vi "final code.vi"() -> ()   [LabVIEW 2018]
uses:
  <vilib>/Analysis/Matrix/Datatypes/RealMatrix.ctl
  <vilib>/Analysis/Matrix/NI_Matrix.lvlib
panel:
  in  "Y":dbl(slide)=1.5703016241299301 scale=1.6..-1.6
  in  "X":dbl(slide)=-1.504382470119522 scale=-1.6..1.6
  out "3D Picture":refnum<vi>(3d-picture)
  in  "stop":bool
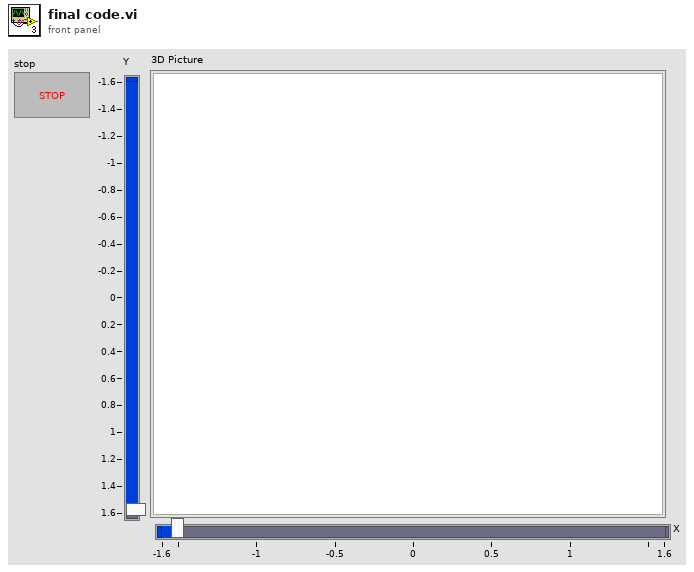
[diagram p1: front panel]
types:
  T1 = cluster{"Line width":sgl, "Line Color":u32, "Axes?":bool}
  T2 = typedef "NI_Matrix.lvlib/RealMatrix.ctl" = dbl[][]
  T3 = cluster{"Theta":dbl, "d":dbl, "a":dbl, "alpha (degrees)":dbl}[]
  T4 = cluster{"Theta":dbl, "d":dbl, "a":dbl, "alpha (degrees)":dbl}
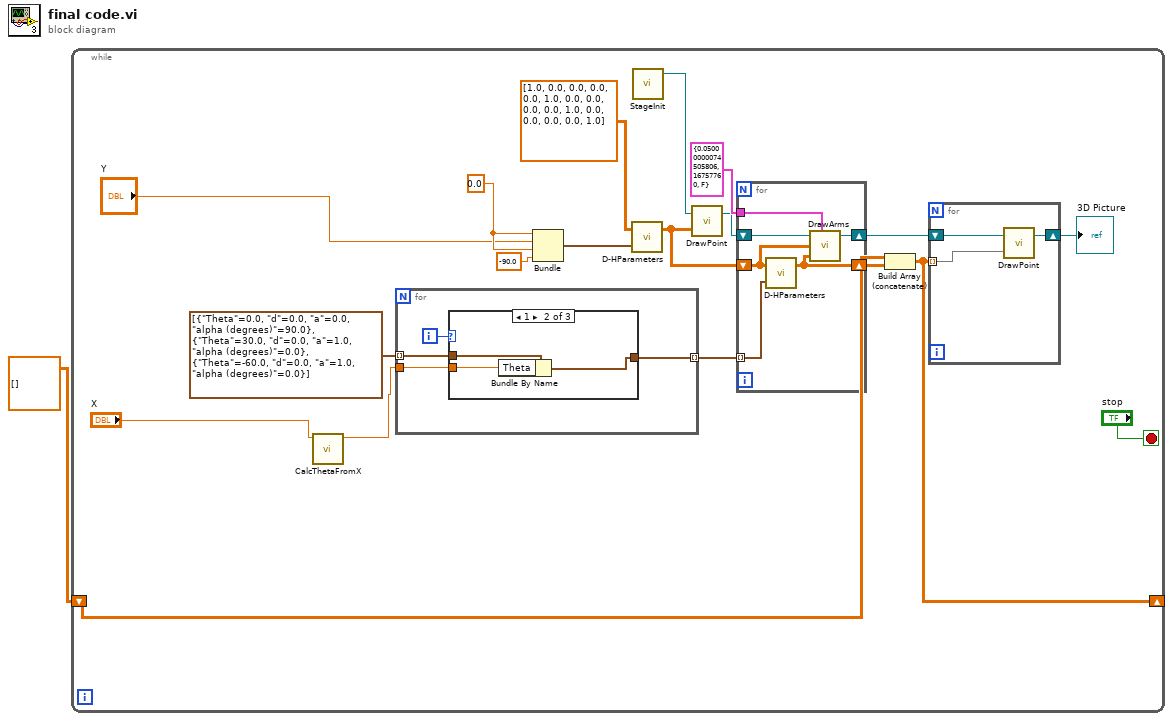
[diagram p0: block diagram]
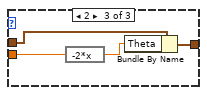
[diagram p3: hidden frame]
diagram:
  n1 = while {
    shift-right: [w19] -> _
    shift-left: dbl[][][] [] -> [w20]
    stop <- "stop" stop-if-true
    w5 = 0.0
    n2 = call "CalcThetaFromX.vi"("X"="X") -> ("Numeric"=w2:dbl)  [unwired: 10 in]
    n3 = for {
      tunnel: T3 [{"Theta"=0.0, "d"=0.0, "a"=0.0, "alpha (degrees)"=90.0}, {"Theta"=30.0, "d"=0.0, "a"=1.0, "alpha (degrees)"=0.0}, {"Theta"=-60.0, "d"=0.0, "a"=1.0, "alpha (degrees)"=0.0}] ("Joints") -> [w32] mode=indexing
      tunnel: [w31] -> w14 mode=indexing
      tunnel: w2 -> [w30]
      i -> [w33]
      n4 = case shown="1" w33 {
        tunnel: w32 -> [w34 w37 w41]
        tunnel: [w34 w36 w40] -> w31
        tunnel: w30 -> [_ w35 w39]
        frame 0, Default {
        }
        frame 1 {
          n5 = Bundle By Name(cluster=w37, "Theta"=w35) -> (w36:T4)
        }
        frame 2 {
          n6 = expression code="-2*x"(w39) -> (w38:dbl)
          n7 = Bundle By Name(cluster=w41, "Theta"=w38) -> (w40:T4)
        }
      }
    }
    n8 = Bundle(w5, "Y"="Y", w5, -90.0) -> (w6:cluster{dbl, "Y":dbl, dbl, dbl})  [unwired: 1 in]
    n9 = call "D-HParameters.vi"("n+1"=w6, "Start"=T2 [[1.0, 0.0, 0.0, 0.0], [0.0, 1.0, 0.0, 0.0], [0.0, 0.0, 1.0, 0.0], [0.0, 0.0, 0.0, 1.0]]) -> ("A x B"=w8:T2)  [unwired: 1 in]
    n10 = call "StageInit.vi"() -> ("Stage out"=w11:refnum<vi>)  [unwired: 4 in, 1 out]
    n11 = call "DrawPoint.vi"("Start"=w8, "Stage in"=w11) -> ("Stage out"=w10:refnum<vi>)  [unwired: 1 in]
    n12 = for {
      shift-right: [w24] -> w15
      shift-left: w8 -> [w25]
      tunnel: w14 -> [w29] mode=indexing
      shift-right: [w27] -> w13
      shift-left: w10 -> [w26]
      tunnel: T1 {"Line width"=0.05, "Line Color"=16757760, "Axes?"=FALSE} ("Params") -> [w28]
      n13 = call "D-HParameters.vi"("n+1"=w29, "Start"=w25) -> ("A x B"=w24:T2)  [unwired: 1 in]
      n14 = call "DrawArms.vi"("Stage in"=w26, "Params"=w28, "Start"=w25, "End"=w24) -> ("Stage out"=w27:refnum<vi>)  [unwired: 2 in, 1 out]
    }
    n15 = Build Array (concatenate)(w20, w15) -> (w19:dbl[][][])
    n16 = for {
      shift-right: [w22] -> w18
      shift-left: w13 -> [w23]
      tunnel: w19 -> [w21] mode=indexing
      n17 = call "DrawPoint.vi"("Start"=w21, "Stage in"=w23) -> ("Stage out"=w22:refnum<vi>)  [unwired: 1 in]
    }
    "3D Picture" <- w18
  }
